vi "Verify Digraph for Supported Datatypes.vi"() -> (3 "test passed":bool)   [LabVIEW 2014]
uses:
  <vilib>/NI/Tag Bus/tag/Data Type.ctl
  GraphViz Mapping Visualizer.lvlib
  <vilib>/NI/Tag Bus/tag/tag descriptor.lvclass
panel:
  out "digraph output":string
  out "node connections with tag names":string[][](array[string])
  out "node connections":string[][](array[string])
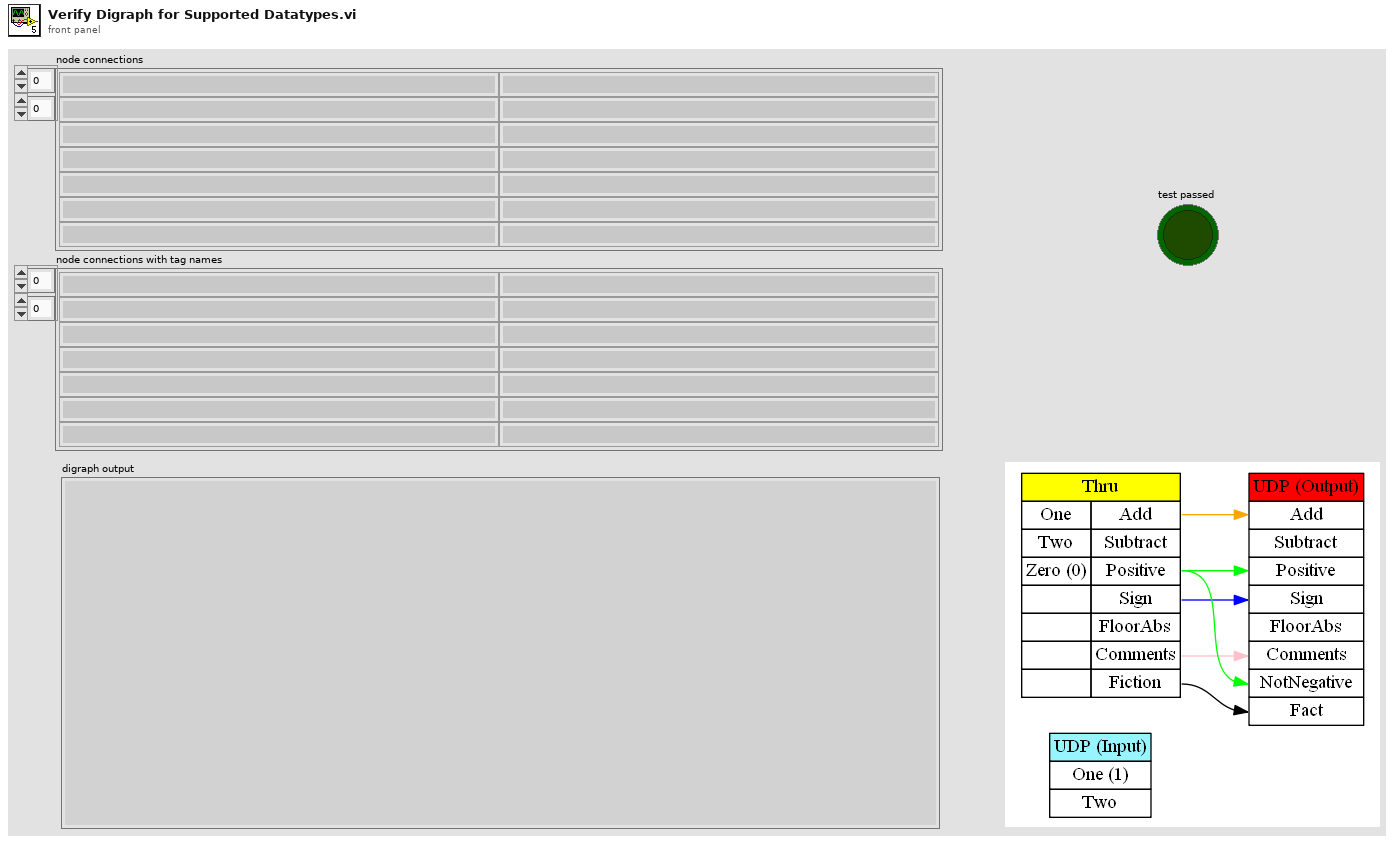
[diagram p1: front panel]
types:
  T1 = cluster{"Instance ID":string, "name":string, "default value string":string, "index":i32}[]
  T2 = typedef "tag bus.lvlib/tag descriptor.lvclass/Data Type.ctl" = enum16{"Double", "Single", "I64", "I32", "I16", "I8", "U64", "U32", "U16", "U8", "Boolean", "String", "Array of Double", "Array of Single", "Array of I64", "Array of I32", "Array of I16", "Array of I8", "Array of U64", "Array of U32", "Array of U16", "Array of U8", "Array of Boolean", "Array of String"}
  T3 = cluster{"name":string, "data type":T2, "writer":string, "readers":string[]}[]
  T4 = cluster{"inbound display strings and indices":cluster{"Instance ID":string, "name":string, "default value string":string, "index":i32}[], "inbound display strings and indices 2":cluster{"Instance ID":string, "name":string, "default value string":string, "index":i32}[]}
  T5 = typedef "GraphViz Mapping Visualizer.lvlib/Channel to Port Pair.ctl" = cluster{"Channel Name":string, "Node:Port":string}
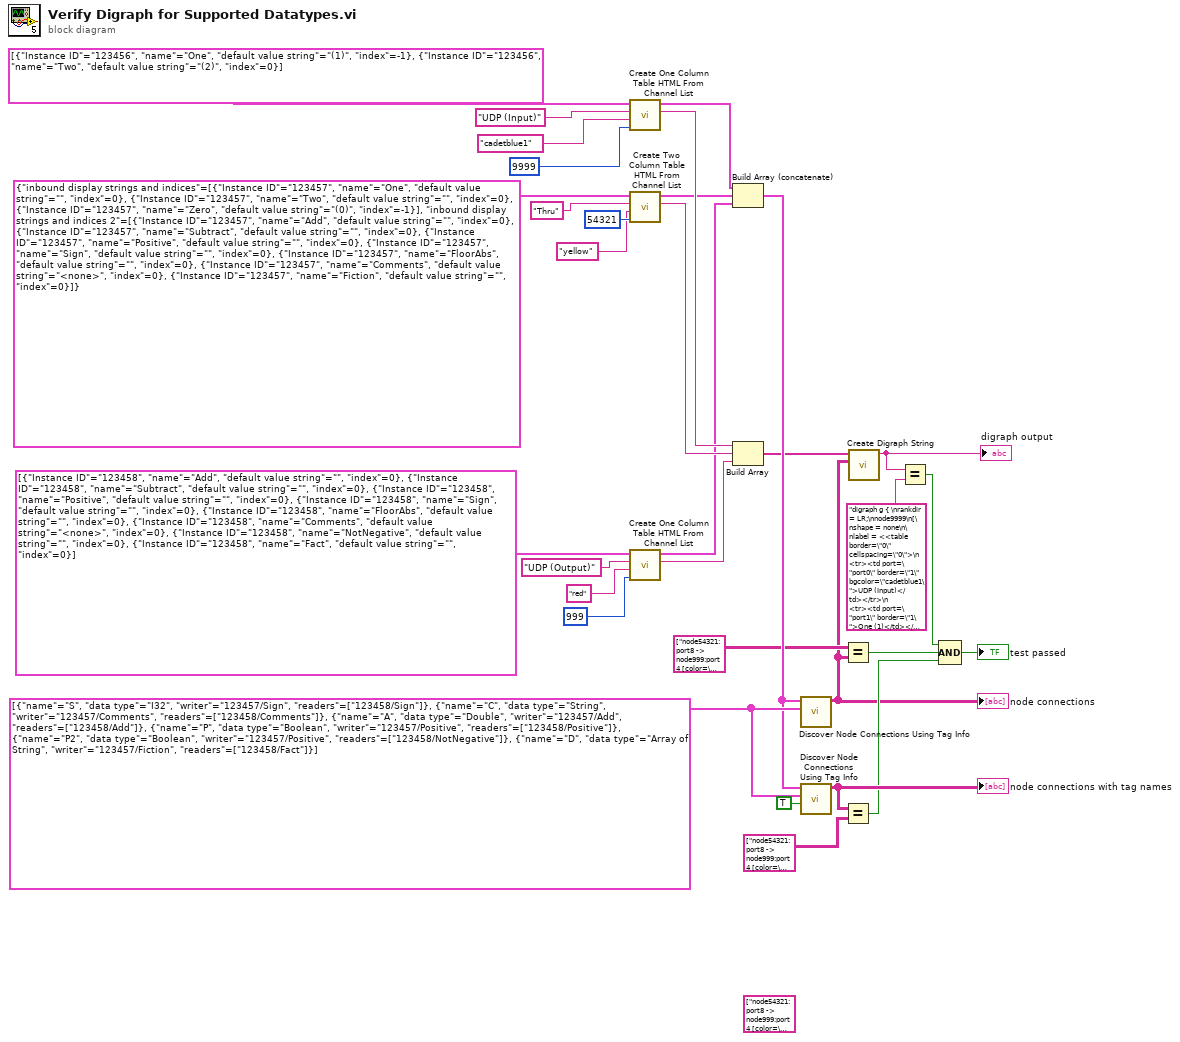
[diagram p0: block diagram]
diagram:
  (unwired) string[][] [["node54321:port8 -> node999:port4 [color=\"blue\"] [label=\"S\"]\r\n"], ["node54321:port12 -> node999:port6 [color=\"pink\"] [label=\"C\"]\r\n"], ["node54321:port2 -> node999:port1 [color=\"orange\"] [label=\"A\"]\r\n"], ["node54321:port6 -> node999:port3 [color=\"green\"] [label=\"P\"]\r\n"], ["node54321:port6 -> node999:port7 [color=\"green\"] [label=\"P2\"]\r\n"], ["node54321:port14 -> node999:port8 [label=\"D\"]\r\n"]] ("node connections 2")
  w26 = T3 [{"name"="S", "data type"=enum."I32", "writer"="123457/Sign", "readers"=["123458/Sign"]}, {"name"="C", "data type"=enum."String", "writer"="123457/Comments", "readers"=["123458/Comments"]}, {"name"="A", "data type"=enum."Double", "writer"="123457/Add", "readers"=["123458/Add"]}, {"name"="P", "data type"=enum."Boolean", "writer"="123457/Positive", "readers"=["123458/Positive"]}, {"name"="P2", "data type"=enum."Boolean", "writer"="123457/Positive", "readers"=["123458/NotNegative"]}, {"name"="D", "data type"=enum."Array of String", "writer"="123457/Fiction", "readers"=["123458/Fact"]}] ("tag info")
  n1 = call "Create One Column Table HTML From Channel List.vi"("Node#"=9999, "Color"="cadetblue1", "Title"="UDP (Input)", "display strings and indices"=T1 [{"Instance ID"="123456", "name"="One", "default value string"="(1)", "index"=-1}, {"Instance ID"="123456", "name"="Two", "default value string"="(2)", "index"=0}]) -> ("Table HTML"=w27:string, "Channel and Node Pairs"=w24:T5[])  [unwired: 6 in]
  n2 = call "Create Two Column Table HTML From Channel List.vi"("Node#"=54321, "Color"="yellow", "Title"="Thru", "process display strings and indices"=T4 {"inbound display strings and indices"=[{"Instance ID"="123457", "name"="One", "default value string"="", "index"=0}, {"Instance ID"="123457", "name"="Two", "default value string"="", "index"=0}, {"Instance ID"="123457", "name"="Zero", "default value string"="(0)", "index"=-1}], "inbound display strings and indices 2"=[{"Instance ID"="123457", "name"="Add", "default value string"="", "index"=0}, {"Instance ID"="123457", "name"="Subtract", "default value string"="", "index"=0}, {"Instance ID"="123457", "name"="Positive", "default value string"="", "index"=0}, {"Instance ID"="123457", "name"="Sign", "default value string"="", "index"=0}, {"Instance ID"="123457", "name"="FloorAbs", "default value string"="", "index"=0}, {"Instance ID"="123457", "name"="Comments", "default value string"="<none>", "index"=0}, {"Instance ID"="123457", "name"="Fiction", "default value string"="", "index"=0}]}) -> ("Table HTML"=w25:string, "Channel and Node Pairs"=w23:T5[])  [unwired: 6 in]
  n3 = call "Create One Column Table HTML From Channel List.vi"("Node#"=999, "Color"="red", "Title"="UDP (Output)", "display strings and indices"=T1 [{"Instance ID"="123458", "name"="Add", "default value string"="", "index"=0}, {"Instance ID"="123458", "name"="Subtract", "default value string"="", "index"=0}, {"Instance ID"="123458", "name"="Positive", "default value string"="", "index"=0}, {"Instance ID"="123458", "name"="Sign", "default value string"="", "index"=0}, {"Instance ID"="123458", "name"="FloorAbs", "default value string"="", "index"=0}, {"Instance ID"="123458", "name"="Comments", "default value string"="<none>", "index"=0}, {"Instance ID"="123458", "name"="NotNegative", "default value string"="", "index"=0}, {"Instance ID"="123458", "name"="Fact", "default value string"="", "index"=0}] ("inbound display strings and indices 2")) -> ("Table HTML"=w6:string, "Channel and Node Pairs"=w18:T5[])  [unwired: 6 in]
  n4 = Build Array (concatenate)(w24, w23, w18) -> (w22:T5[])
  n5 = Build Array(w27, w25, w6) -> (w4:string[])
  n6 = call "Discover Node Connections Using Tag Info.vi"("tag info"=w26, "channel and node pairs"=w22) -> ("node connections"=w5:string[][])  [unwired: 9 in]
  "node connections" <- w5
  n7 = call "Discover Node Connections Using Tag Info.vi"("Show Tag Labels?"=TRUE, "tag info"=w26, "channel and node pairs"=w22) -> ("node connections"=w11:string[][])  [unwired: 8 in]
  "node connections with tag names" <- w11
  n8 = Equal?(x=string[][] [["node54321:port8 -> node999:port4 [color=\"blue\"]\r\n"], ["node54321:port12 -> node999:port6 [color=\"pink\"]\r\n"], ["node54321:port2 -> node999:port1 [color=\"orange\"]\r\n"], ["node54321:port6 -> node999:port3 [color=\"green\"]\r\n"], ["node54321:port6 -> node999:port7 [color=\"green\"]\r\n"], ["node54321:port14 -> node999:port8\r\n"]] ("node connections"), y=w5) -> (x = y?=w9:bool)
  n9 = Equal?(x=w11, y=string[][] [["node54321:port8 -> node999:port4 [color=\"blue\"] [label=\"S\"]\r\n"], ["node54321:port12 -> node999:port6 [color=\"pink\"] [label=\"C\"]\r\n"], ["node54321:port2 -> node999:port1 [color=\"orange\"] [label=\"A\"]\r\n"], ["node54321:port6 -> node999:port3 [color=\"green\"] [label=\"P\"]\r\n"], ["node54321:port6 -> node999:port7 [color=\"green\"] [label=\"P2\"]\r\n"], ["node54321:port14 -> node999:port8 [label=\"D\"]\r\n"]] ("node connections 2")) -> (x = y?=w8:bool)
  n10 = call "Create Digraph String.vi"("node connections"=w5, "tables html"=w4) -> ("digraph output"=w3:string)  [unwired: 9 in]
  "digraph output" <- w3
  n11 = Equal?(x=w3, y="digraph g { \nrankdir = LR;\nnode9999\n[\nshape = none\n\nlabel = <<table border=\"0\" cellspacing=\"0\">\n                    <tr><td port=\"port0\" border=\"1\" bgcolor=\"cadetblue1\">UDP (Input)</td></tr>\n                    <tr><td port=\"port1\" border=\"1\">One (1)</td></tr>\n                    <tr><td port=\"port2\" border=\"1\">Two</td></tr>\n</table>>\n]\nnode54321\n[\nshape = none\n\nlabel = <<table border=\"0\" cellspacing=\"0\">\n                    <tr><td COLSPAN=\"2\" port=\"port0\" border=\"1\" bgcolor=\"yellow\">Thru</td></tr>\n                    <tr><td port=\"port1\" border=\"1\">One</td><td port=\"port2\" border=\"1\">Add</td></tr>\n                    <tr><td port=\"port3\" border=\"1\">Two</td><td port=\"port4\" border=\"1\">Subtract</td></tr>\n                    <tr><td port=\"port5\" border=\"1\">Zero (0)</td><td port=\"port6\" border=\"1\">Positive</td></tr>\n                    <tr><td port=\"port7\" border=\"1\"></td><td port=\"port8\" border=\"1\">Sign</td></tr>\n                    <tr><td port=\"port9\" border=\"1\"></td><td port=\"port10\" border=\"1\">FloorAbs</td></tr>\n                    <tr><td port=\"port11\" border=\"1\"></td><td port=\"port12\" border=\"1\">Comments</td></tr>\n                    <tr><td port=\"port13\" border=\"1\"></td><td port=\"port14\" border=\"1\">Fiction</td></tr>\n</table>>\n]\nnode999\n[\nshape = none\n\nlabel = <<table border=\"0\" cellspacing=\"0\">\n                    <tr><td port=\"port0\" border=\"1\" bgcolor=\"red\">UDP (Output)</td></tr>\n                    <tr><td port=\"port1\" border=\"1\">Add</td></tr>\n                    <tr><td port=\"port2\" border=\"1\">Subtract</td></tr>\n                    <tr><td port=\"port3\" border=\"1\">Positive</td></tr>\n                    <tr><td port=\"port4\" border=\"1\">Sign</td></tr>\n                    <tr><td port=\"port5\" border=\"1\">FloorAbs</td></tr>\n                    <tr><td port=\"port6\" border=\"1\">Comments</td></tr>\n                    <tr><td port=\"port7\" border=\"1\">NotNegative</td></tr>\n                    <tr><td port=\"port8\" border=\"1\">Fact</td></tr>\n</table>>\n]\nnode54321:port8 -> node999:port4 [color=\"blue\"]\r\nnode54321:port12 -> node999:port6 [color=\"pink\"]\r\nnode54321:port2 -> node999:port1 [color=\"orange\"]\r\nnode54321:port6 -> node999:port3 [color=\"green\"]\r\nnode54321:port6 -> node999:port7 [color=\"green\"]\r\nnode54321:port14 -> node999:port8\r\n}" ("digraph output")) -> (x = y?=w1:bool)
  n12 = Compound Arithmetic op=AND(w1, w9, w8) -> (→"test passed":bool)
